vi "Convert Actuator Setpoint.vi"(8 "error in (no error)":errorcluster, 11 "Model in":refnum<class "Model.lvclass">) -> (0 "error out":errorcluster, 3 "Model out":refnum<class "Model.lvclass">)   [LabVIEW 2015, in "Model.lvclass"]
uses:
  Model.lvclass
  Model.lvclass/Model.ctl
  Calculators/Actuator To Cylinder Forces/Actuator To Cylinder Forces.lvclass
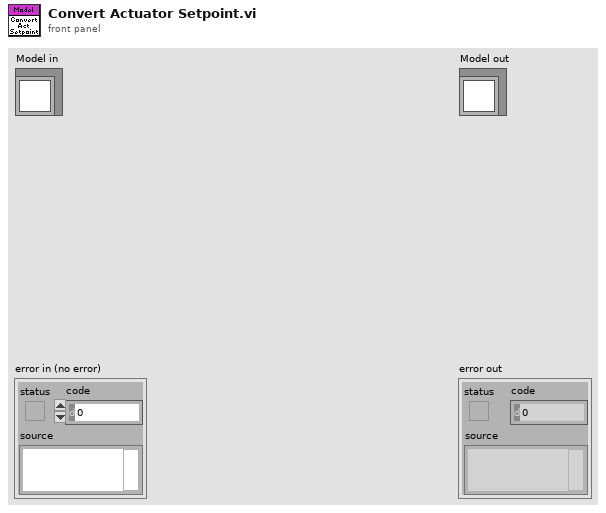
[diagram p1: front panel]
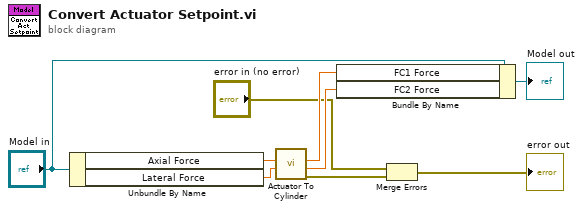
[diagram p0: block diagram]
diagram:
  n1 = Unbundle By Name("Model in") -> ("Axial Force"=w9:dbl, "Lateral Force"=w8:dbl)
  n2 = call "Actuator To Cylinder.vi"("Lateral Force"=w8, "Axial Force"=w9) -> ("error out"=w3:errorcluster, "FC2 Value"=w5:dbl, "FC1 Value"=w6:dbl)  [unwired: 6 in, 1 out]
  n3 = Bundle By Name(cluster="Model in", "FC1 Force"=w6, "FC2 Force"=w5) -> (→"Model out":refnum<class "Model.lvclass">)
  n4 = Merge Errors("error in (no error)", w3) -> (→"error out":errorcluster)
